vi "CMD_Vision.vi"(1 "Line":string) -> (0 "Done":bool)   [LabVIEW 2017, in "Apple script.lvlib"]
uses:
  Apple script.lvlib
  Robot Global Data.vi
panel:
  in  "Parameters":i32[](array[numeric])=[0, 1]
  in  "Subcommands":string[](array[string])=["harvest", "for"]
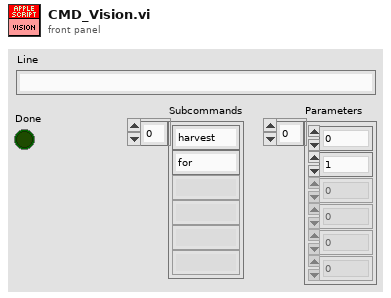
[diagram p1: front panel]
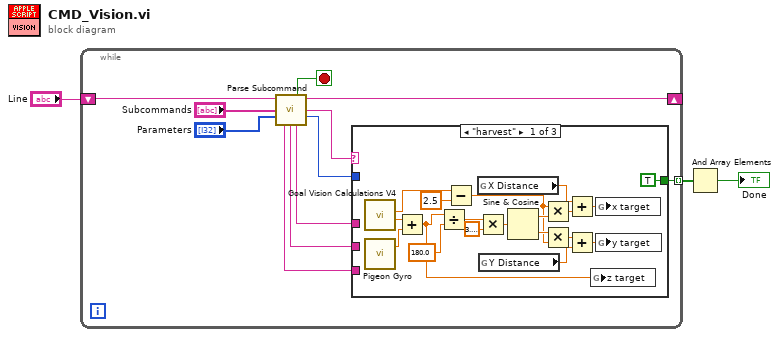
[diagram p0: block diagram]
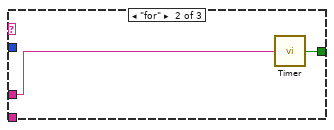
[diagram p2: hidden frame]
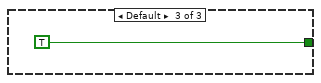
[diagram p3: hidden frame]
diagram:
  n1 = while {
    shift-right: [w11] -> _
    shift-left: "Line" -> [w14]
    tunnel: [w4] -> w2 mode=indexing
    stop <- w10 stop-if-true
    n2 = call "Parse Subcommand.vi"("Text In"=w14, "Subcommands"="Subcommands", "Parameters"="Parameters") -> ("Done"=w10:bool, "Text Out"=w11:string, "Subcommand"=w9:string, "# of Parameters"=w8:i32, "Parameter 3"=w5:string, "Parameter 2"=w6:string, "Parameter 1"=w7:string)  [unwired: 6 in]
    n3 = case shown="\"harvest\"" w9 {
      tunnel: w8 -> [_ _ _]
      tunnel: w7 -> [_ w34 _]
      tunnel: w6 -> [_ _ _]
      tunnel: w5 -> [_ _ _]
      tunnel: [TRUE w35 TRUE] -> w4
      frame "harvest" {
        n4 = call "Goal Vision Calculations V4.vi"() -> ("Angle"=w32:dbl, "distance ft"=w18:dbl)  [unwired: 9 in]
        n5 = call "Pigeon Gyro.vi"() -> ("YPR.Yaw"=w31:dbl)  [unwired: 2 in, 1 out]
        n6 = Add(x=w32, y=w31) -> (x+y=w15:dbl)
        n7 = Divide(x=w15, y=180.0) -> (x/y=w19:dbl)
        n8 = Subtract(x=w18, y=2.5) -> (x-y=w21:dbl)
        n9 = global read "Robot Global Data.vi" "X Distance"() -> (w23:dbl)
        n10 = Multiply(x=w19, y=3.141592653589793) -> (x*y=w20:dbl)
        n11 = global read "Robot Global Data.vi" "Y Distance"() -> (w28:dbl)
        n12 = Sine & Cosine(0:w20) -> (1:w25:dbl, 2:w30:dbl)
        n13 = Multiply(x=w21, y=w25) -> (x*y=w24:dbl)
        n14 = Multiply(x=w30, y=w21) -> (x*y=w29:dbl)
        n15 = Add(x=w23, y=w24) -> (x+y=w26:dbl)
        n16 = Add(x=w29, y=w28) -> (x+y=w27:dbl)
        n17 = global write "Robot Global Data.vi" "z target"(w15) -> ()
        n18 = global write "Robot Global Data.vi" "x target"(w26) -> ()
        n19 = global write "Robot Global Data.vi" "y target"(w27) -> ()
      }
      frame "for" {
        n20 = call "Timer.vi"("Seconds (string)"=w34) -> ("Done"=w35:bool)
      }
      frame Default {
      }
    }
  }
  n21 = And Array Elements(Boolean array=w2) -> (logical AND=→"Done":bool)
